vi "Calibrate Drive.vi"   [LabVIEW 2014]
uses:
  Global Variables.vi
types:
  T1 = typedef "WPI_AnalogChannelDevRef.ctl" = cluster{"DevStatus":errorcluster, "Controller":T2, "Analog Channel":T3}
  T2 = typedef "FPGA_TypedefAnalogModule.ctl" = enum16{"Controller 1"}
  T3 = typedef "FPGA_AIChannel.ctl" = enum8{"AI 0", "AI 1", "AI 2", "AI 3", "AI MXP 0", "AI MXP 1", "AI MXP 2", "AI MXP 3", "Invalid"}
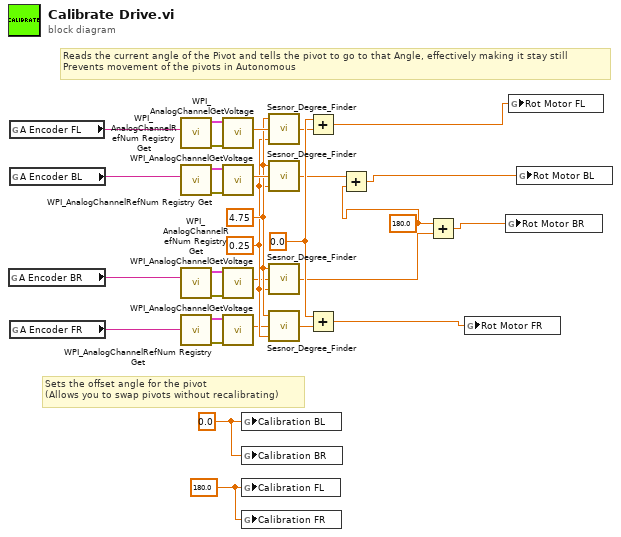
[diagram p0: block diagram]
diagram:
  w1 = 180.0 ("Calibration FL")
  w2 = 0.0 ("Calibration BL")
  w11 = 180.0 ("x")
  w30 = 0.0
  w16 = 0.25
  w17 = 4.75
  # "Reads the current angle of the Pivot and tells the pivot to go to that Angle, effectively making it stay still\nPrevents movement of the pivots in Autonomous"
  # "Sets the offset angle for the pivot\n(Allows you to swap pivots without recalibrating)"
  n1 = global read "Global Variables.vi" "A Encoder BR"() -> (w8:string)
  n2 = global read "Global Variables.vi" "A Encoder FL"() -> (w10:string)
  n3 = global read "Global Variables.vi" "A Encoder BL"() -> (w9:string)
  n4 = global read "Global Variables.vi" "A Encoder FR"() -> (w7:string)
  n5 = call <vilib>:"WPI_AnalogChannelRefNum Registry Get.vi"("refnum name"=w10) -> ("error out"=w25:errorcluster, "AIDeviceRef"=w24:T1)  [unwired: 9 in]
  n6 = call <vilib>:"WPI_AnalogChannelRefNum Registry Get.vi"("refnum name"=w9) -> ("error out"=w28:errorcluster, "AIDeviceRef"=w29:T1)  [unwired: 9 in]
  n7 = call <vilib>:"WPI_AnalogChannelRefNum Registry Get.vi"("refnum name"=w8) -> ("error out"=w27:errorcluster, "AIDeviceRef"=w26:T1)  [unwired: 9 in]
  n8 = call <vilib>:"WPI_AnalogChannelRefNum Registry Get.vi"("refnum name"=w7) -> ("error out"=w23:errorcluster, "AIDeviceRef"=w22:T1)  [unwired: 9 in]
  n9 = call <vilib>:"WPI_AnalogChannelGetVoltage.vi"("error in (no error)"=w25, "AIDeviceRef"=w24) -> ("Voltage"=w20:dbl)  [unwired: 7 in, 2 out]
  n10 = call <vilib>:"WPI_AnalogChannelGetVoltage.vi"("error in (no error)"=w28, "AIDeviceRef"=w29) -> ("Voltage"=w19:dbl)  [unwired: 7 in, 2 out]
  n11 = call <vilib>:"WPI_AnalogChannelGetVoltage.vi"("error in (no error)"=w27, "AIDeviceRef"=w26) -> ("Voltage"=w15:dbl)  [unwired: 7 in, 2 out]
  n12 = call <vilib>:"WPI_AnalogChannelGetVoltage.vi"("error in (no error)"=w23, "AIDeviceRef"=w22) -> ("Voltage"=w14:dbl)  [unwired: 7 in, 2 out]
  n13 = global write "Global Variables.vi" "Calibration BL"(w2) -> ()
  n14 = global write "Global Variables.vi" "Calibration BR"(w2) -> ()
  n15 = global write "Global Variables.vi" "Calibration FL"(w1) -> ()
  n16 = global write "Global Variables.vi" "Calibration FR"(w1) -> ()
  n17 = call "Sesnor_Degree_Finder.vi"("Minimum Volts"=w16, "Voltage"=w20, "Max Volts"=w17) -> ("Degrees"=w21:dbl)
  n18 = call "Sesnor_Degree_Finder.vi"("Minimum Volts"=w16, "Voltage"=w19, "Max Volts"=w17) -> ("Degrees"=w18:dbl)
  n19 = call "Sesnor_Degree_Finder.vi"("Minimum Volts"=w16, "Voltage"=w15, "Max Volts"=w17) -> ("Degrees"=w13:dbl)
  n20 = call "Sesnor_Degree_Finder.vi"("Minimum Volts"=w16, "Voltage"=w14, "Max Volts"=w17) -> ("Degrees"=w12:dbl)
  n21 = Add(x=w30, y=w21) -> (x+y=w6:dbl)
  n22 = Add(x=w30, y=w12) -> (x+y=w3:dbl)
  n23 = Add(x=w18, y=w11) -> (x+y=w5:dbl)
  n24 = Add(x=w11, y=w13) -> (x+y=w4:dbl)
  n25 = global write "Global Variables.vi" "Rot Motor FR"(w3) -> ()
  n26 = global write "Global Variables.vi" "Rot Motor BR"(w4) -> ()
  n27 = global write "Global Variables.vi" "Rot Motor FL"(w6) -> ()
  n28 = global write "Global Variables.vi" "Rot Motor BL"(w5) -> ()
